vi "Conv_GyroDegrees_Heading.vi"(10 "GyroDegrees":dbl) -> (2 "HeadingDegrees":dbl)   [LabVIEW 2019, in "PathExecution_Library.lvlib"]
doc: "Convert angle (radians) to heading (+/- PI ) (radians)\nNOTE: gyro increments clockwise. Headings increment counterclockwise"
uses:
  PathExecution_Library.lvlib
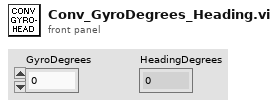
[diagram p1: front panel]
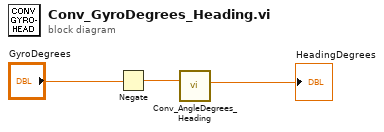
[diagram p0: block diagram]
diagram:
  n1 = Negate(x="GyroDegrees") -> (-x=w2:dbl)
  n2 = call "Conv_AngleDegrees_Heading.vi"("Degrees"=w2) -> ("HeadingDegrees"=→"HeadingDegrees":dbl)  [unwired: 10 in]
